vi "ex_createNewChannelsTDMS.vi"(0 "DAQmx Task":T2, 1 "tdms file in":refnum<k34>, 2 "append info in":T1, 5 "signals":waveform(dbl)[](array[waveform]), 7 "file params":T6 {"Flags"."time preference" items=["Absolute", "Relative"]; "Flags"."x_columns" items=["None", "One", "Multiple"]; "origin time" format="%<%X\n%x>T"}, 9 "File path":path, 10 "is first call":bool, 11 "error in (no error)":errorcluster, 12 "Comment":string, 13 "Description":string, 14 "write file properties":bool) -> (3 "append info out":T1, 4 "tdms file out":refnum<k34>, 6 "bytes written":i32, 8 "error out":errorcluster)   [LabVIEW 2020]
uses:
  express output/ExFileWriteBlock.llb/ex_WriteFileParams.ctl
  express input/ExFileReadBlock.llb/ex_ReadFileParams.ctl
  ex_EditUserDefinedProperties/ex_userdefproperties.ctl
  ExFile.llb/ex_userDefProperty.ctl
  ex_EditUserDefinedProperties/usiDataType.ctl
  ExFile.llb/ex_propertySource.ctl
  Platform/express/TDMExpress.llb/ex_appendInfoTDM.ctl
  Platform/storage/lvStorage.llb/_wf_attributes.ctl
  Platform/storage/lvStorage.llb/_stringsToBeTranslated.ctl
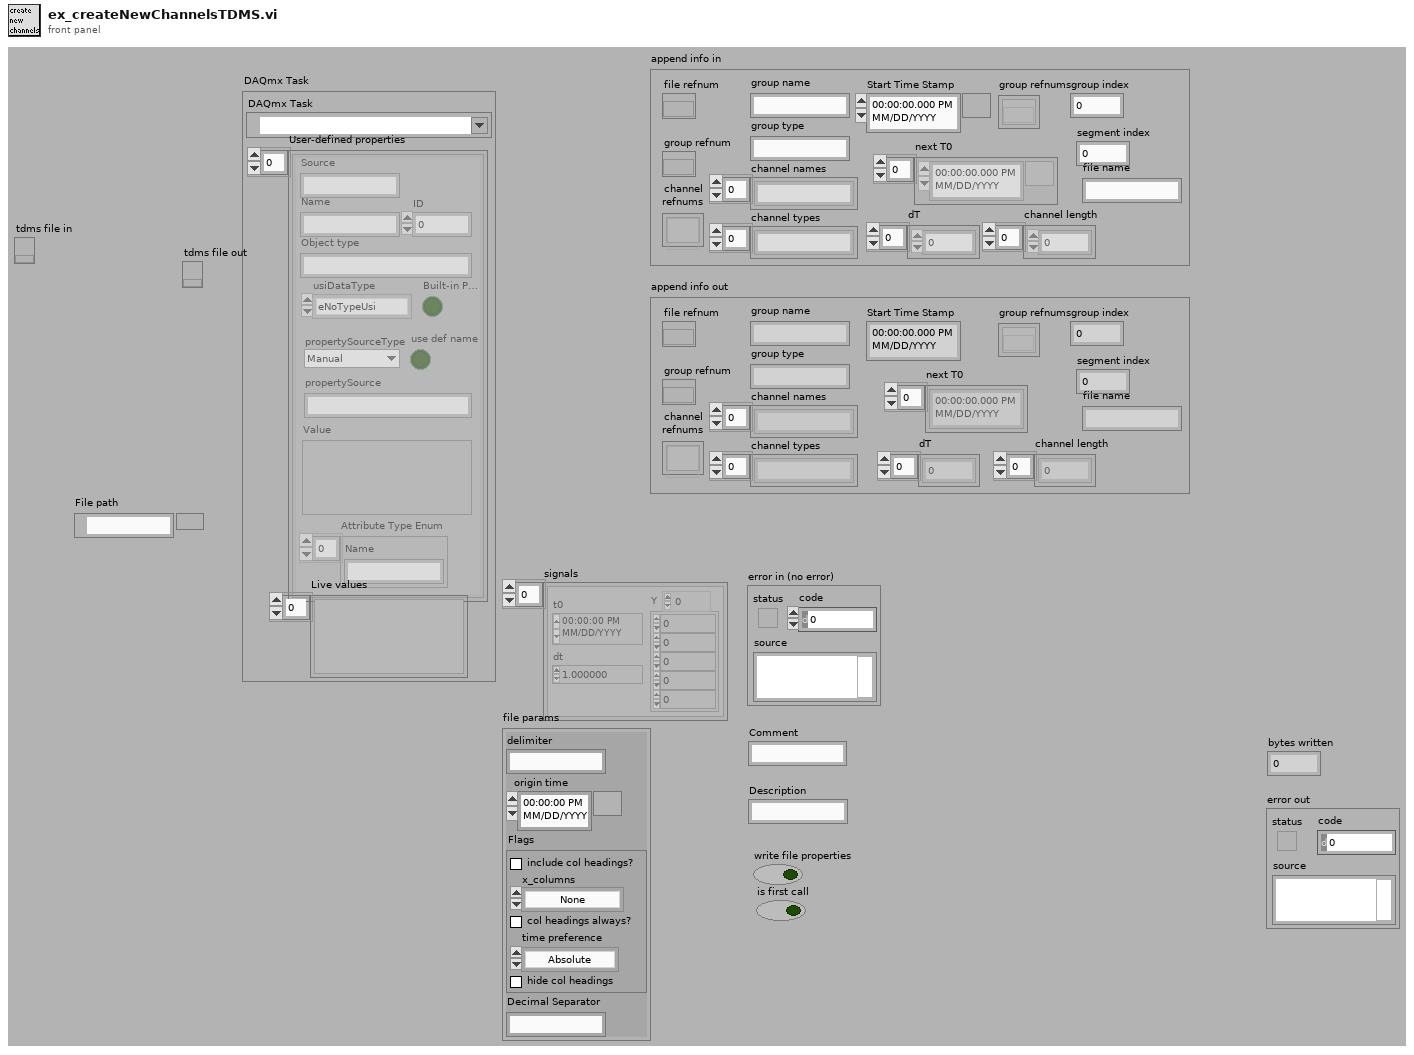
[diagram p1: front panel]
types:
  T1 = typedef "ex_appendInfoTDM.ctl" = cluster{"channel\nrefnums":refnum<k20>[], "channel names":string[], "channel types":string[], "file refnum":refnum<k20>, "group refnum":refnum<k20>, "group name":string, "group type":string, "next T0":timestamp[], "dT":dbl[], "Start Time Stamp":timestamp, "channel length":u32[], "group index":u32, "group refnums":refnum<k20>[], "file name":string, "segment index":u32}
  T2 = typedef "ex_userdefproperties.ctl" = cluster{"DAQmx Task":refnum<k21>, "User-defined properties":T3[], "Live values":variant[]}
  T3 = typedef "ex_userDefProperty.ctl" = cluster{"Name":string, "Object type":string, "usiDataType":T4, "propertySourceType":T5, "propertySource":string, "Value":variant, "ID":i32, "use def name":bool, "Source":string, "Built-in Prop":bool, "Attribute Type Enum":string[]}
  T4 = typedef "usiDataType.ctl" = enum16{"eNoTypeUsi", "eInt8Usi", "eInt16Usi", "eInt32Usi", "eInt64Usi", "eUInt8Usi", "eUInt16Usi", "eUInt32Usi", "eUInt64Usi", "eFloat32Usi", "eFloat64Usi", "- 0", "- 1", "- 2", "- 3", "- 4", "- 5", "- 6", "- 7", "- 8", "- 9", "eString8Usi", "eString16Usi", "eStringUsi", "eEnumUsi", "- 10", "- 11", "- 12", "- 13", "- 14", "eTimeUsi", "- 15", "- 16", "- 17", "- 18", "- 19", "- 20", "- 21", "- 22", "- 23", "eInstanceUsi", "eStoreUsi"}
  T5 = typedef "ex_propertySource.ctl" = enum16{"Manual", "System", "DAQmx Channel", "Terminal", "Ignore"}
  T6 = typedef "ex_WriteFileParams.ctl" = cluster{"delimiter":string, "origin time":timestamp, "Flags":T7, "Decimal Separator":string}
  T7 = typedef "ex_ReadFileParams.ctl" = cluster{"include col headings?":bool, "x_columns":u16, "col headings always?":bool, "time preference":u16, "hide col headings":bool}
  T8 = typedef "_stringsToBeTranslated.ctl" = enum16{"Properties", "View as icon", "query all data", "Load Storage VI parameters into memory", "Dynamically assign format", "Enumerated type", "Time stamp", "Configure", "Size to text", "Untitled", "storage refnum", "Load waveform data", "TDM (...)", "LVM (...)", "CSV (...)", "DYN (...)", "WrittenByLabVIEW", "TDMS", "out"}
  T9 = typedef "_wf_attributes.ctl" = enum16{"t0", "dt", "X_Name", "X_Unit", "x0", "abs/rel", "nPoints", "file_timestamp", "xcolumns"}
  T10 = typedef "ex_TdmData.ctl" = cluster{"New file":bool, "New header":bool, "File properties":T11[], "Header properties":T11[], "Signal properties":T11[][], "Signal values":waveform(dbl)[]}
  T11 = typedef "ex_TdmProperty.ctl" = cluster{"Name":string, "Type":T4, "Value":variant}
  T12 = cluster{"Start Timestamp":timestamp, "Timestamp":timestamp, "Relative Time?":bool, "X Dimension":string, "Signal Name":string, "Y Units":string, "X0":timestamp, "dX":dbl, "nPoints":i32}[]
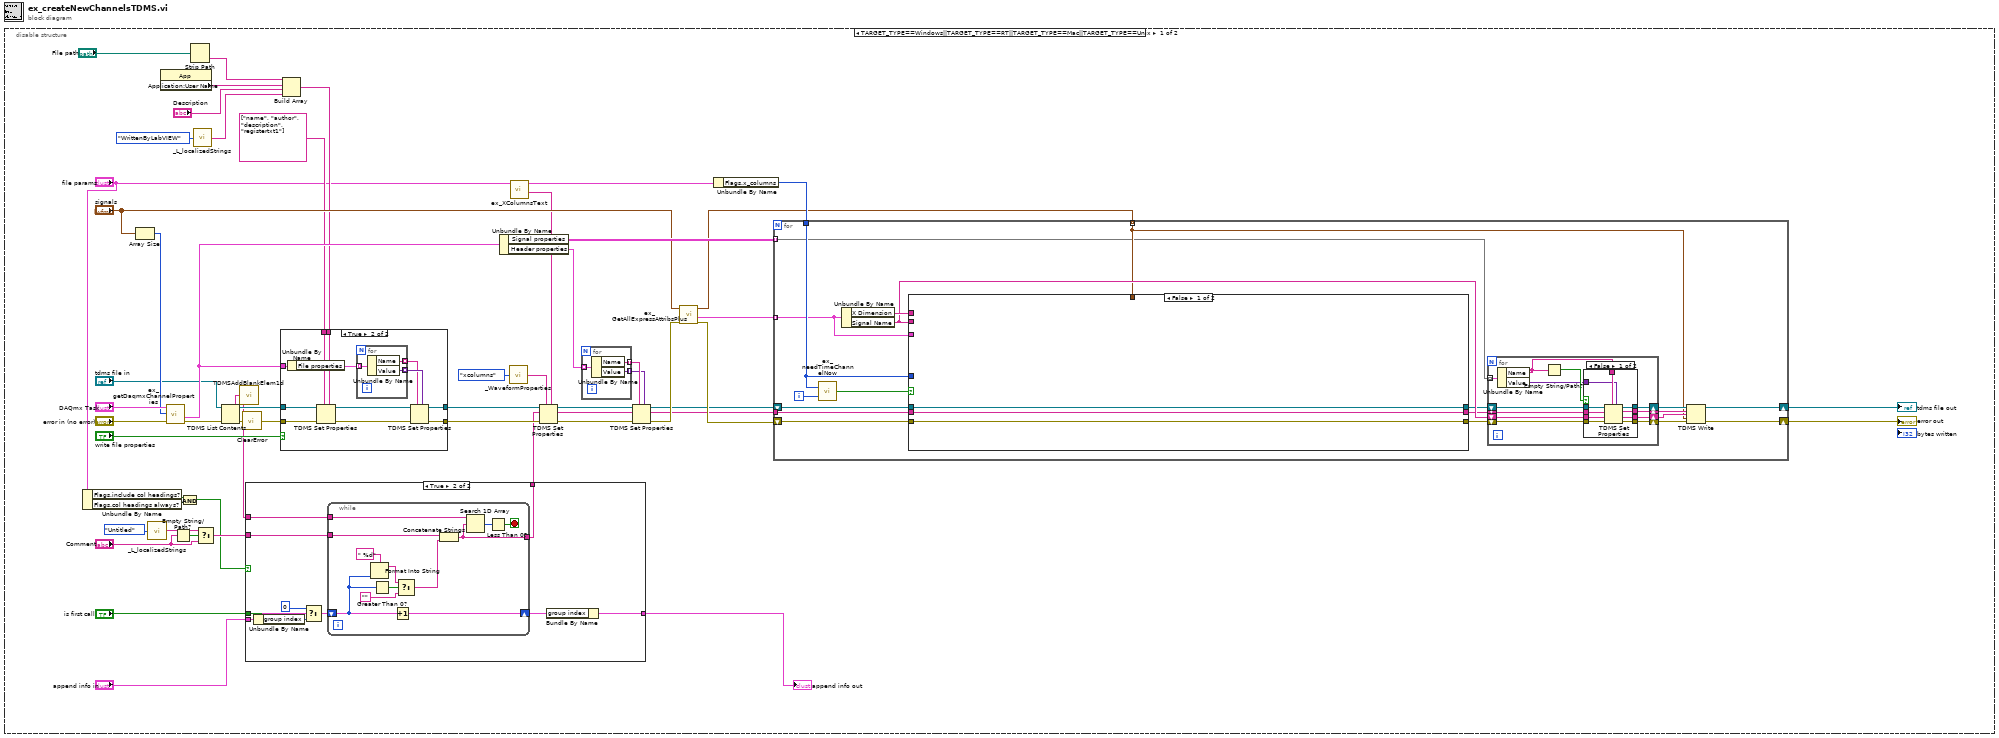
[diagram p0: block diagram]
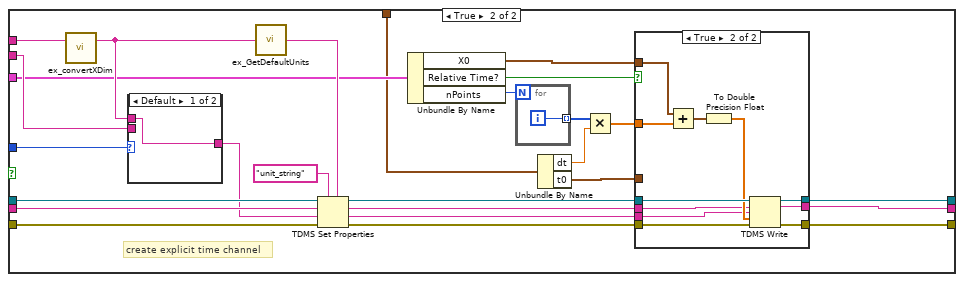
[diagram p5: hidden frame]
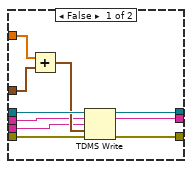
[diagram p6: hidden frame]
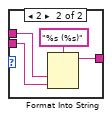
[diagram p7: hidden frame]
diagram:
  n1 = disable-structure shown="TARGET_TYPE==Windows||TARGET_TYPE==RT||TARGET_TYPE==Mac||TARGET_TYPE==Unix" {
    frame condition #0 (active) {
      n2 = Unbundle By Name("file params") -> ("Flags.include col headings?"=w18:bool, "Flags.col headings always?"=w19:bool)
      n3 = Array Size(array="signals") -> (size(s)=w46:i32)
      n4 = call "_L_localizedStrings.vi"(1:_stringsToBeTranslated."Untitled") -> (0:w5:string)
      n5 = property class="App"() -> ("Application:User Name"=w24:string)  [unwired: 2 in, 2 out]
      n6 = call "ex_getDaqmxChannelProperties.vi"("error in (no error)"="error in (no error)", "Number of channels (if no DAQmx task available)"=w46, "task"="DAQmx Task") -> ("error out"=w13:errorcluster, "all properties"=w50:T10)  [unwired: 1 in, 2 out]
      n7 = Empty String/Path?(string/path="Comment") -> (empty?=w7:bool)
      n8 = And(x=w18, y=w19) -> (x .and. y?=w3:bool)
      n9 = Strip Path(path="File path") -> (name=w25:string)  [unwired: 1 out]
      n10 = call "_L_localizedStrings.vi"(1:_stringsToBeTranslated."WrittenByLabVIEW") -> (0:w22:string)
      n11 = Select(t=w5, s=w7, f="Comment") -> (s? t:f=w4:string)
      n12 = TDMS List Contents(4:w13, 7:"tdms file in") -> (0:w1:errorcluster, 2:w2:string[], 3:w11:refnum<k34>)  [unwired: 2 out]
      n13 = call "TDMSAddBlankElem1d.vi"("input string array"=w2) -> ("output string array with blank element at the beginning"=w9:string[])
      n14 = call "ClearError.vi"("error in (no error)"=w1) -> ("error out"=w12:errorcluster)
      n15 = case shown="True" w3 {
        tunnel: [w58 w68] -> w21
        tunnel: "append info in" -> [w57 w67]
        tunnel: [w57 w66] -> w16
        tunnel: "is first call" -> [_ w65]
        tunnel: w9 -> [_ w61]
        tunnel: w4 -> [w58 w59]
        frame False {
        }
        frame True {
          n16 = Unbundle By Name(w67) -> ("group index"=w63:u32)
          n17 = Select(t=u32 0 ("group index"), s=w65, f=w63) -> (s? t:f=w62:u32)
          n18 = while {
            tunnel: [w73] -> w68
            shift-right: [w74] -> w60
            shift-left: w62 -> [w75]
            tunnel: w61 -> [w72]
            tunnel: w59 -> [w69]
            stop <- w70 stop-if-true
            n19 = Format Into String(format string=" %d", w75) -> (resulting string=w77:string)  [unwired: 2 in, 1 out]
            n20 = Greater Than 0?(x=w75) -> (x > 0?=w80:bool)
            n21 = Increment(x=w75) -> (x+1=w74:u32)
            n22 = Select(t=w77, s=w80, f="") -> (s? t:f=w76:string)
            n23 = Concatenate Strings(w69, w76) -> (w73:string)
            n24 = Search 1D Array(1D array=w72, element=w73) -> (index of element=w71:i32)  [unwired: 1 out]
            n25 = Less Than 0?(x=w71) -> (x < 0?=w70:bool)
          }
          n26 = Bundle By Name(cluster=w67, "group index"=w60) -> (w66:T1)
        }
      }
      "append info out" <- w16
      n27 = Build Array(w25, w24, "Description", w22) -> (w43:string[])
      n28 = case shown="True" "write file properties" {
        tunnel: w50 -> [_ w94]
        tunnel: w12 -> [w81 w93]
        tunnel: w43 -> [_ w92]
        tunnel: string[] ["name", "author", "description", "registertxt1"] -> [_ w91]
        tunnel: [w81 w85] -> w41
        tunnel: [w82 w84] -> w40
        tunnel: w11 -> [w82 w83]
        frame False {
        }
        frame True {
          n29 = Unbundle By Name(w94) -> ("File properties"=w90:T11[])
          n30 = TDMS Set Properties(5:w92, 7:w91, 8:w93, 11:w83) -> (0:w88:errorcluster, 3:w89:refnum<k34>)  [unwired: 4 out]
          n31 = for {
            tunnel: w90 -> [w97] mode=indexing
            tunnel: [w96] -> w86 mode=indexing
            tunnel: [w95] -> w87 mode=indexing
            n32 = Unbundle By Name(w97) -> ("Name"=w96:string, "Value"=w95:variant)
          }
          n33 = TDMS Set Properties(5:w87, 7:w86, 8:w88, 11:w89) -> (0:w85:errorcluster, 3:w84:refnum<k34>)  [unwired: 4 out]
        }
      }
      n34 = Unbundle By Name(w50) -> ("Signal properties"=w49:T11[][], "Header properties"=w37:T11[])
      n35 = call "_WaveformProperties.vi"("Property"=_wf_attributes."xcolumns") -> ("Name"=w39:string)
      n36 = call "ex_XColumnsText.vi"("file info in"="file params") -> ("xcolumns"=w38:string, "file info out"=w55:T6)  [unwired: 5 out]
      n37 = TDMS Set Properties(5:w38, 7:w39, 8:w41, 10:w21, 11:w40) -> (0:w34:errorcluster, 2:w36:string, 3:w35:refnum<k34>)  [unwired: 2 out]
      n38 = for {
        tunnel: w37 -> [w100] mode=indexing
        tunnel: [w99] -> w33 mode=indexing
        tunnel: [w98] -> w32 mode=indexing
        n39 = Unbundle By Name(w100) -> ("Name"=w99:string, "Value"=w98:variant)
      }
      n40 = TDMS Set Properties(5:w32, 7:w33, 8:w34, 10:w36, 11:w35) -> (0:w31:errorcluster, 2:w30:string, 3:w29:refnum<k34>)  [unwired: 2 out]
      n41 = call "ex_GetAllExpressAttribsPlus.vi"("error in"=w31, "Signals in"="signals") -> ("error out"=w48:errorcluster, "All Express Wave Attributes Plus"=w54:T12, "Signals out"=w26:waveform(dbl)[])  [unwired: 7 out]
      n42 = Unbundle By Name(w55) -> ("Flags.x_columns"=w56:u16)
      n43 = for {
        tunnel: w54 -> [w109] mode=indexing
        shift-right: [w105] -> w27
        shift-left: w48 -> [w120]
        tunnel: w56 -> [w115]
        tunnel: w49 -> [w101] mode=indexing
        tunnel: w30 -> [w114]
        shift-right: [w106] -> w28
        shift-left: w29 -> [w118]
        tunnel: w26 -> [w102] mode=indexing
        i -> [w119]
        n44 = call "ex_needTimeChannelNow.vi"("index"=w119, "x_columns"=w115) -> ("need time channel NOW !!!!"=w116:bool)
        n45 = Unbundle By Name(w109) -> ("X Dimension"=w117:string, "Signal Name"=w112:string)
        n46 = case shown="False" w116 {
          tunnel: w118 -> [w147 w170]
          tunnel: w120 -> [w149 w171]
          tunnel: [w149 w154] -> w113
          tunnel: w112 -> [_ w175]
          tunnel: w117 -> [_ w173]
          tunnel: w115 -> [_ w174]
          tunnel: w114 -> [w148 w169]
          tunnel: [w148 w151] -> w111
          tunnel: [w147 w155] -> w110
          tunnel: w109 -> [_ w156]
          tunnel: w102 -> [_ w150]
          frame False {
          }
          frame True {
            # "create explicit time channel"
            n47 = call "ex_convertXDim.vi"("x_dimension in"=w173) -> ("x_dimension out"=w172:string)  [unwired: 1 in, 1 out]
            n48 = case shown="Default" w174 {
              tunnel: [w198 w201] -> w168
              tunnel: w172 -> [w198 w200]
              tunnel: w175 -> [_ w199]
              frame Default {
              }
              frame 2 {
                n49 = Format Into String(format string="%s (%s)", w200, w199) -> (resulting string=w201:string)  [unwired: 2 in, 1 out]
              }
            }
            n50 = call "ex_GetDefaultUnits.vi"("dimension"=w172) -> ("default units"=w166:string)
            n51 = TDMS Set Properties(5:w166, 7:"unit_string" ("Property name"), 8:w171, 9:w168, 10:w169, 11:w170) -> (0:w158:errorcluster, 1:w153:string, 2:w152:string, 3:w157:refnum<k34>)
            n52 = Unbundle By Name(w156) -> ("X0"=w164:timestamp, "Relative Time?"=w162:bool, "nPoints"=w159:i32)
            n53 = for {
              N: w159 -> [_]
              tunnel: [w197] -> w160 mode=indexing
              i -> [w197]
            }
            n54 = Unbundle By Name(w150) -> ("dt"=w161:dbl, "t0"=w165:timestamp)
            n55 = Multiply(x=w160, y=w161) -> (x*y=w163:dbl[])
            n56 = case shown="True" w162 {
              tunnel: w163 -> [w185 w195]
              tunnel: w164 -> [_ w196]
              tunnel: w165 -> [w184 _]
              tunnel: w157 -> [w183 w190]
              tunnel: w158 -> [w182 w191]
              tunnel: [w181 w192] -> w154
              tunnel: [w180 w193] -> w155
              tunnel: w153 -> [w178 w187]
              tunnel: w152 -> [w177 w188]
              tunnel: [w176 w186] -> w151
              frame False {
                n57 = Add(x=w185, y=w184) -> (x+y=w179:timestamp[])
                n58 = TDMS Write(0:w183, 5:w177, 7:w178, 9:w179, 11:w182) -> (4:w180:refnum<k34>, 6:w176:string, 15:w181:errorcluster)  [unwired: 1 in, 1 out]
              }
              frame True {
                n59 = Add(x=w196, y=w195) -> (x+y=w194:timestamp[])
                n60 = To Double Precision Float(number=w194) -> (double precision float=w189:dbl[])
                n61 = TDMS Write(0:w190, 5:w188, 7:w187, 9:w189, 11:w191) -> (4:w193:refnum<k34>, 6:w186:string, 15:w192:errorcluster)  [unwired: 1 in, 1 out]
              }
            }
          }
        }
        n62 = for {
          shift-right: [w127] -> w107
          shift-left: w113 -> [w132]
          shift-right: [w125] -> w103
          shift-left: w112 -> [w131]
          shift-right: [w126] -> w104
          shift-left: w111 -> [w130]
          shift-right: [w128] -> w108
          shift-left: w110 -> [w129]
          tunnel: w101 -> [w124] mode=indexing
          n63 = Unbundle By Name(w124) -> ("Name"=w122:string, "Value"=w121:variant)
          n64 = Empty String/Path?(string/path=w122) -> (empty?=w123:bool)
          n65 = case shown="False" w123 {
            tunnel: w132 -> [w142 w143]
            tunnel: w131 -> [w141 w144]
            tunnel: w130 -> [w140 w145]
            tunnel: w129 -> [w139 w146]
            tunnel: [w138 w146] -> w128
            tunnel: [w137 w143] -> w127
            tunnel: [w136 w145] -> w126
            tunnel: [w135 w144] -> w125
            tunnel: w122 -> [w134 _]
            tunnel: w121 -> [w133 _]
            frame False {
              n66 = TDMS Set Properties(5:w133, 7:w134, 8:w142, 9:w141, 10:w140, 11:w139) -> (0:w137:errorcluster, 1:w135:string, 2:w136:string, 3:w138:refnum<k34>)
            }
            frame True {
            }
          }
        }
        n67 = TDMS Write(0:w108, 5:w104, 7:w103, 9:w102, 11:w107) -> (4:w106:refnum<k34>, 15:w105:errorcluster)  [unwired: 1 in, 2 out]
      }
      "error out" <- w27
      "tdms file out" <- w28
    }
    frame condition #1 {
    }
  }
